vi "controls test.vi"() -> ()   [LabVIEW 2020]
panel:
  out "concatenated string":string
  out "choose side RING output":u16(ring) items=["LEFT", "RIGHT"]
  in  "choose side":u16(ring) items=["LEFT", "RIGHT"]
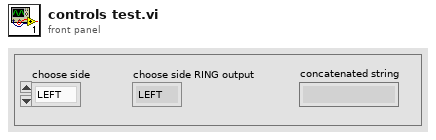
[diagram p1: front panel]
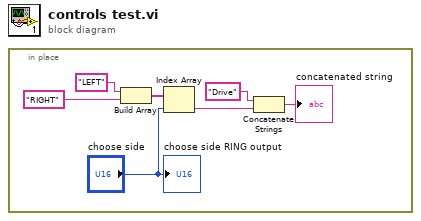
[diagram p0: block diagram]
diagram:
  n1 = in-place {
    n2 = Build Array("LEFT" ("string"), "RIGHT" ("string")) -> (w4:string[])
    n3 = Index Array(array=w4, index="choose side") -> (element=w3:string)
    n4 = Concatenate Strings("Drive" ("string"), w3) -> (→"concatenated string":string)
    "choose side RING output" <- "choose side"
  }
